vi "Unmarshal.vi"(8 "error in (no error)":errorcluster, 10 "Buffer":u8[](array[numeric]), 11 "int32 in":refnum<class "packed.lvclass">) -> (0 "error out":errorcluster, 2 "Buffer Count":i32=8, 3 "int32 out":refnum<class "packed.lvclass">)   [LabVIEW 2020, in "Protobuf RAW.lvlib" / "packed.lvclass"]
uses:
  packed.lvclass
  packed.lvclass/packed.ctl
  Scalar Encoder/Scalar Type.lvclass
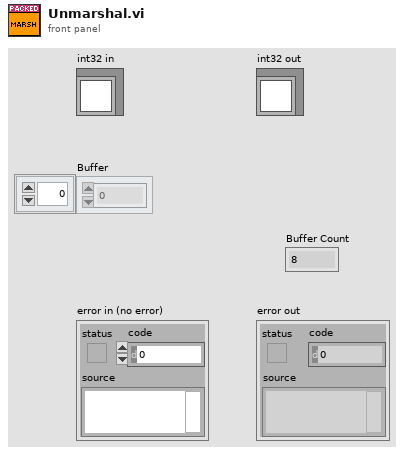
[diagram p1: front panel]
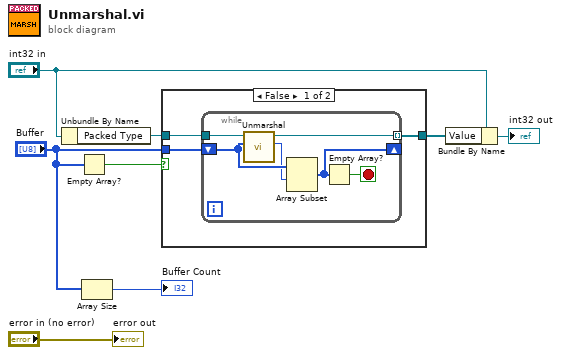
[diagram p0: block diagram]
diagram:
  n1 = Unbundle By Name("int32 in") -> ("Packed Type"=w5:refnum<class "Scalar Type.lvclass">)
  n2 = Empty Array?(array="Buffer") -> (empty?=w3:bool)
  n3 = Array Size(array="Buffer") -> (size(s)=→"Buffer Count":i32)
  n4 = case shown="False" w3 {
    tunnel: w5 -> [w11 _]
    tunnel: [w10 _] -> w4
    tunnel: "Buffer" -> [w9 _]
    frame False {
      n5 = while {
        tunnel: w11 -> [w17]
        tunnel: [w16] -> w10 mode=indexing
        shift-right: [w12] -> _
        shift-left: w9 -> [w15]
        stop <- w13 stop-if-true
        n6 = call-dynamic "Unmarshal.vi"("Buffer"=w15, "Type Serializer in"=w17) -> ("Buffer Count"=w14:i32, "Type Serializer out"=w16:refnum<class "Scalar Type.lvclass">)  [unwired: 7 in, 1 out]
        n7 = Array Subset(array=w15, index=w14) -> (w12:u8[])  [unwired: 1 in]
        n8 = Empty Array?(array=w12) -> (empty?=w13:bool)
      }
    }
    frame True {
    }
  }
  n9 = Bundle By Name(cluster="int32 in", "Value"=w4) -> (→"int32 out":refnum<class "packed.lvclass">)
  "error out" <- "error in (no error)"
